vi "SeCrTs-TC_Scale.vi"(8 "error in (no error)":errorcluster, 10 "TC":T1(array[cluster]), 11 "Refnum in":refnum<k21>) -> (0 "error out":errorcluster, 3 "Refnum out":refnum<k21>)   [LabVIEW 2022 SP3]
uses:
  <vilib>/DAQmx/create/channels.llb/DAQmx Create Channel (AI-Temperature-Thermocouple).vi
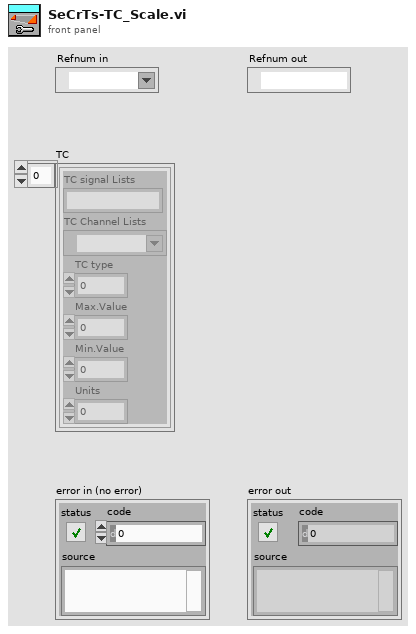
[diagram p1: front panel]
types:
  T1 = cluster{"TC signal Lists":string, "TC Channel Lists":tag, "TC type":i32, "Max.Value":dbl, "Min.Value":dbl, "Units":i32}[]
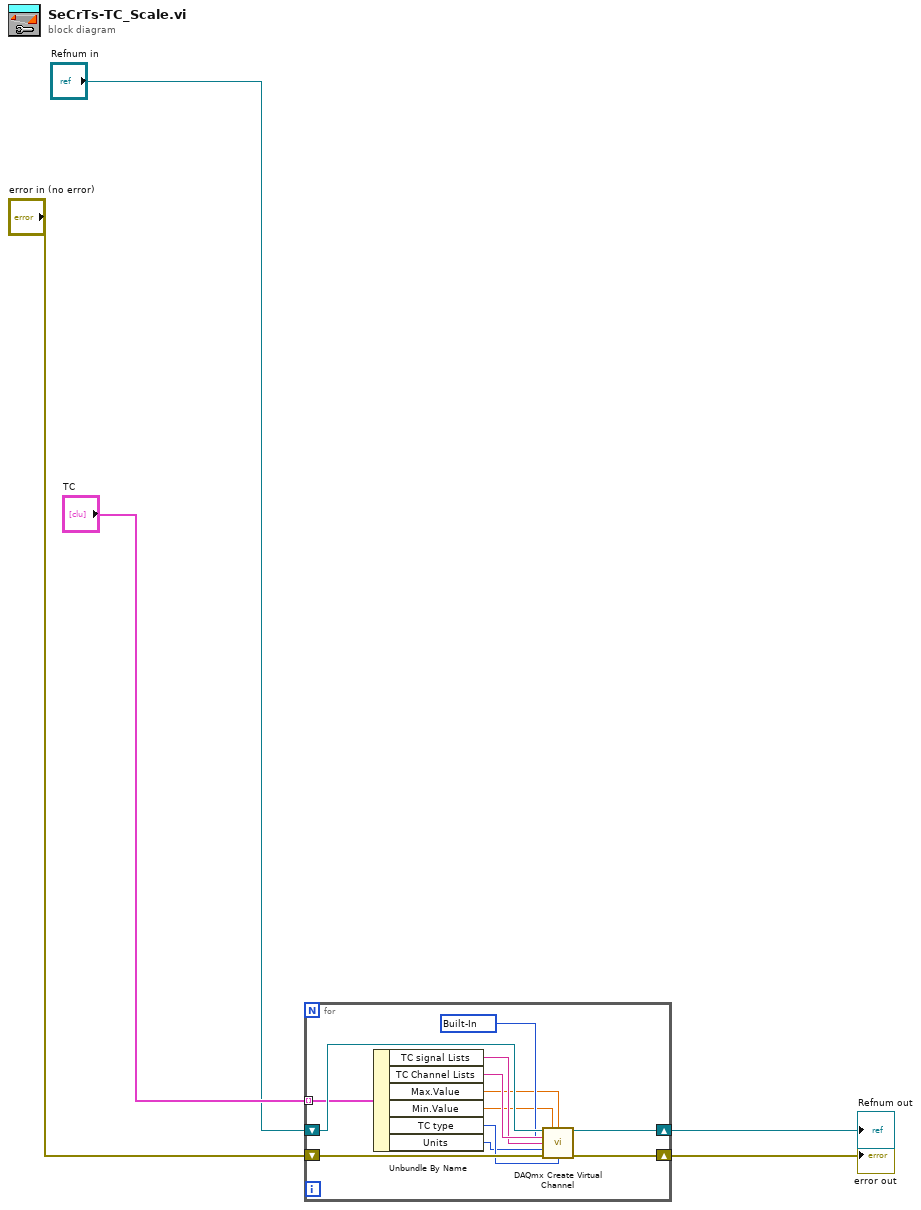
[diagram p0: block diagram]
diagram:
  n1 = for {
    shift-right: [w16] -> w2
    shift-left: "Refnum in" -> [w17]
    shift-right: [w15] -> w1
    shift-left: "error in (no error)" -> [w12]
    tunnel: "TC" -> [w11] mode=indexing
    w10 = 10200 items=["Built-In"=10200, "Constant Value"=10116, "Channel"=10113] ("cjc source")
    n2 = Unbundle By Name(w11) -> ("TC signal Lists"=w13:string, "TC Channel Lists"=w14:tag, "Max.Value"=w9:dbl, "Min.Value"=w8:dbl, "TC type"=w7:i32, "Units"=w6:i32)
    n3 = call-poly <vilib>:"DAQmx Create Virtual Channel.vi"("task in"=w17, "maximum value"=w8, "minimum value"=w9, "physical channels"=w14, "cjc source"=w10, "name to assign"=w13, "units"=w6, "error in"=w12, "thermocouple type"=w7) -> ("task out"=w16:refnum<k21>, "error out"=w15:errorcluster)  [unwired: 5 in]
  }
  "Refnum out" <- w2
  "error out" <- w1
